vi "WriteToFile-v3.vi"(0 "Refnum in":refnum<k34>, 1 "Group Name":string, 2 "IO Names":string[](array[string]), 5 "rt fifo":refnum<k33>, 9 "Write?":bool, 11 "error in (no error)":errorcluster, 12 "ConstNames":string[](array[string]), 13 "ConstValues":dbl[](array[numeric])) -> (4 "Refnum out":refnum<k34>, 10 "Writing to file":bool, 15 "error out":errorcluster)   [LabVIEW 2018]
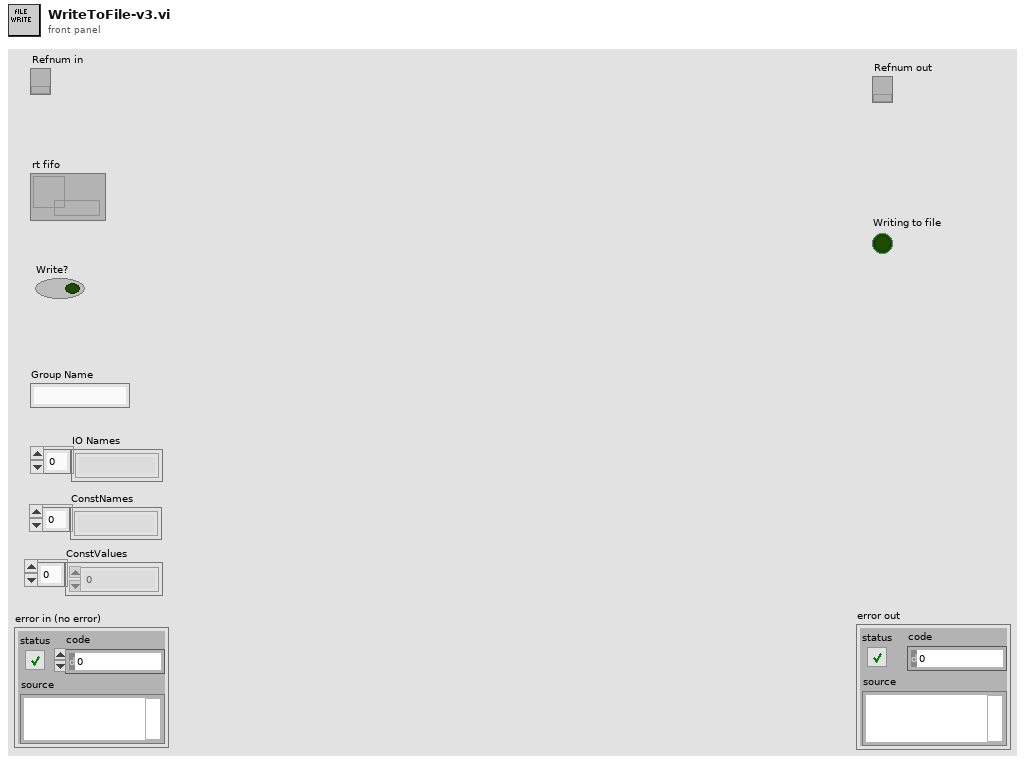
[diagram p1: front panel]
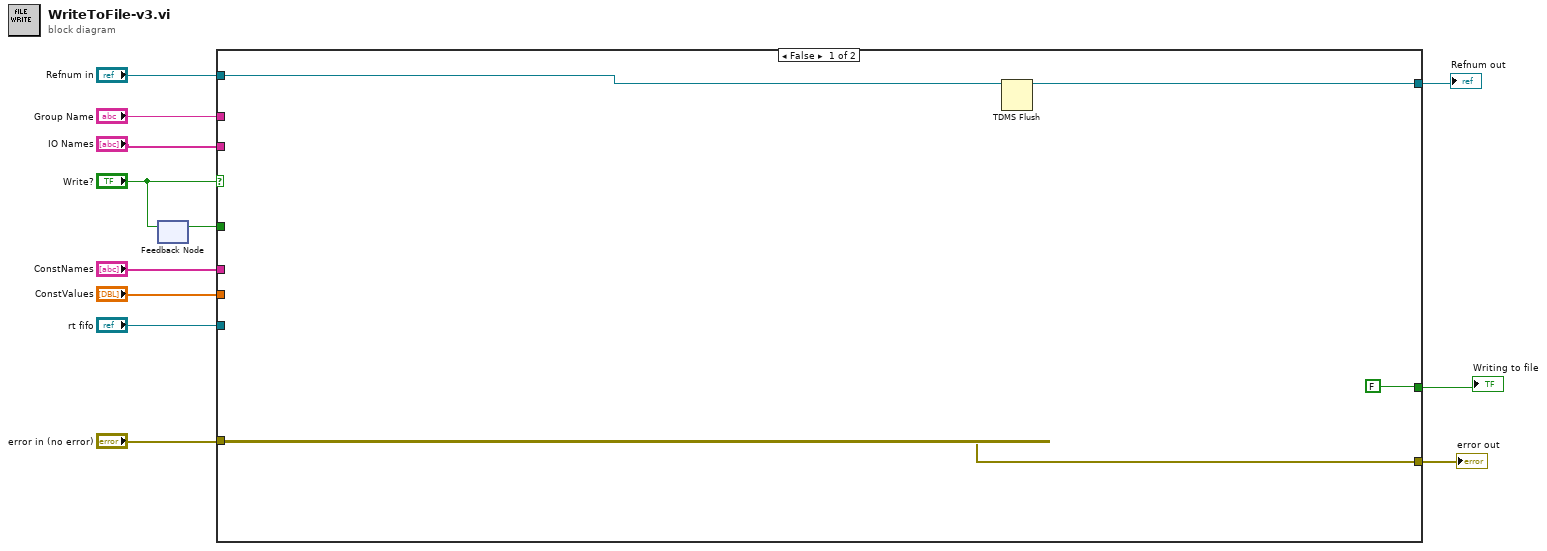
[diagram p0: block diagram]
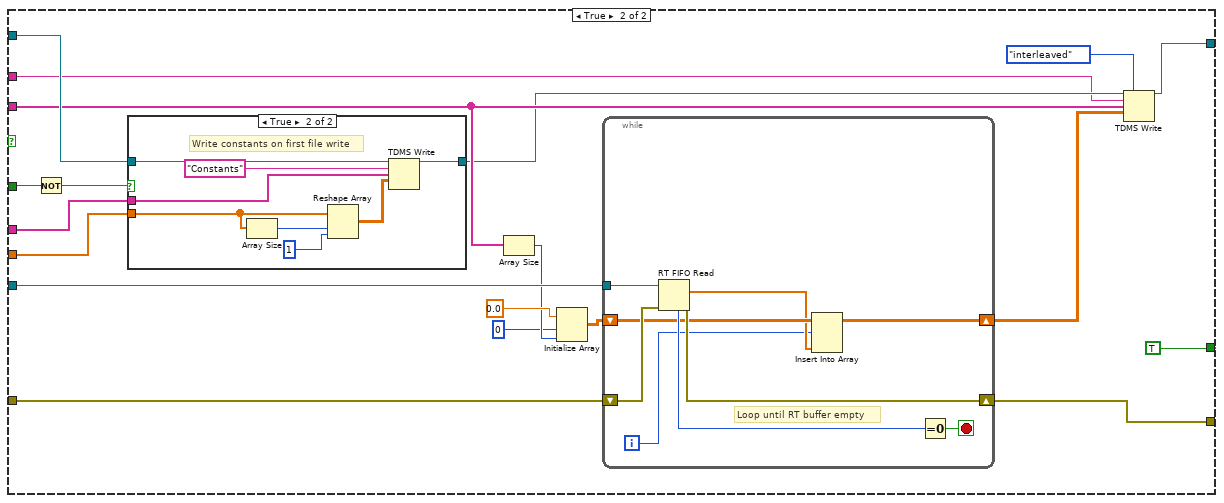
[diagram p2: hidden frame]
diagram:
  n1 = feedback #1() -> (w3:bool)  [unwired: 1 in]
  n2 = feedback-in #1("Write?") -> ()
  n3 = case shown="False" "Write?" {
    tunnel: "Refnum in" -> [w14 w31]
    tunnel: [w13 w21] -> w9
    tunnel: [w15 w32] -> w10
    tunnel: "IO Names" -> [_ w26]
    tunnel: "Group Name" -> [_ w22]
    tunnel: [FALSE ("Writing to file") TRUE ("Writing to file")] -> w7
    tunnel: "rt fifo" -> [_ w33]
    tunnel: "error in (no error)" -> [w15 w34]
    tunnel: w3 -> [_ w30]
    tunnel: "ConstNames" -> [_ w28]
    tunnel: "ConstValues" -> [_ w27]
    frame False {
      n4 = TDMS Flush(7:w14) -> (3:w13:refnum<k34>)  [unwired: 1 in, 1 out]
    }
    frame True {
      n5 = Not(x=w30) -> (.not. x?=w29:bool)
      n6 = case shown="True" w29 {
        tunnel: w31 -> [w36 w44]
        tunnel: [w36 w43] -> w23
        tunnel: w28 -> [_ w39]
        tunnel: w27 -> [_ w38]
        frame False {
        }
        frame True {
          # "Write constants on first file write"
          n7 = Array Size(array=w38) -> (size(s)=w40:i32)
          n8 = Reshape Array(w38, w40, 1) -> (w37:dbl[][])
          n9 = TDMS Write(0:w44, 5:"Constants" ("group name in (Untitled)"), 7:w39, 9:w37) -> (4:w43:refnum<k34>)  [unwired: 2 in, 3 out]
        }
      }
      n10 = Array Size(array=w26) -> (size(s)=w20:i32)
      n11 = Initialize Array(0.0 ("element"), 0 ("dimension size"), w20) -> (w24:dbl[][])
      n12 = while {
        tunnel: w33 -> [w53]
        shift-right: [w51] -> w32
        shift-left: w34 -> [w52]
        shift-right: [w47] -> w18
        shift-left: w24 -> [w48]
        i -> [w45]
        stop <- w50 stop-if-true
        # "Loop until RT buffer empty"
        n13 = RT FIFO Read(0:w53, 3:w52) -> (7:w49:u32, 9:w46:dbl[], 11:w51:errorcluster)  [unwired: 2 in, 2 out]
        n14 = Insert Into Array(array=w48, index (row)=w45, new element=w46) -> (w47:dbl[][])  [unwired: 1 in]
        n15 = Equal To 0?(x=w49) -> (x = 0?=w50:bool)
      }
      n16 = TDMS Write(0:w23, 1:enum16{"decimated", "interleaved"}."interleaved" ("data layout (0:decimated)"), 5:w22, 7:w26, 9:w18) -> (4:w21:refnum<k34>)  [unwired: 1 in, 3 out]
    }
  }
  "error out" <- w10
  "Refnum out" <- w9
  "Writing to file" <- w7
